vi "Destroy Texture.vi"(8 "error in (no error)":errorcluster, 11 "Texture Name":string) -> (0 "error out":errorcluster)   [LabVIEW 2021, in "Resource Manager.lvclass"]
uses:
  Resource Manager.lvclass
  Texture/Texture.lvclass
  Resource Manager.lvclass/Resource Manager.ctl
  Globals.vi
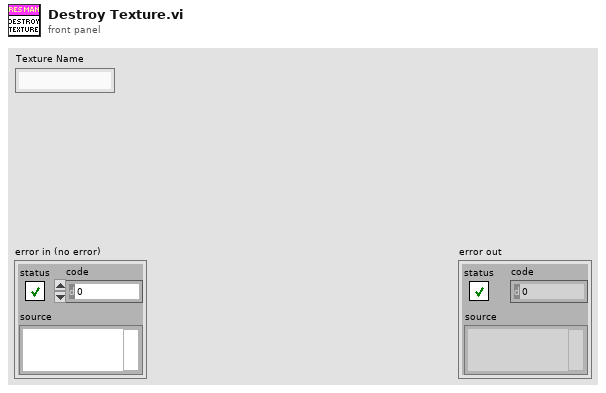
[diagram p1: front panel]
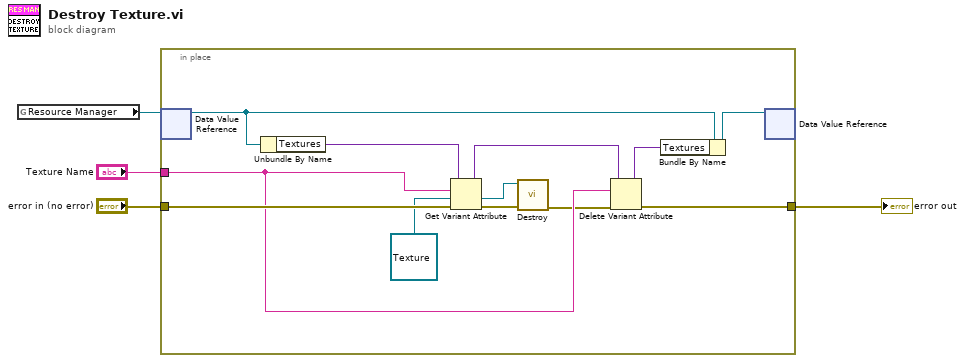
[diagram p0: block diagram]
diagram:
  n1 = global read "Globals.vi" "Resource Manager"() -> (w1:refnum<data-value>)
  n2 = in-place {
    in-place-border: "error in (no error)" -> [w15]
    in-place-border: [w12] -> w3
    in-place-border: "Texture Name" -> [w10]
    n3 = in-place-dvr #1(w1) -> (w6:refnum<class "Resource Manager.lvclass">)  [unwired: 1 out]
    n4 = Unbundle By Name(w6) -> ("Textures"=w16:variant)
    n5 = Get Variant Attribute(Variant=w16, name=w10, default value (empty Variant)=refnum<class "Texture.lvclass"> refnum ("Texture in"), error in=w15) -> (duplicate Variant=w13:variant, value=w8:refnum<class "Texture.lvclass">, error out=w9:errorcluster)  [unwired: 1 out]
    n6 = call "Destroy.vi"("error in (no error)"=w9, "Texture in"=w8) -> ("error out"=w7:errorcluster)  [unwired: 9 in]
    n7 = Delete Variant Attribute(4:w7, 6:w10, 7:w13) -> (0:w12:errorcluster, 3:w11:variant)  [unwired: 1 out]
    n8 = Bundle By Name(cluster=w6, "Textures"=w11) -> (w5:refnum<class "Resource Manager.lvclass">)
    n9 = in-place-dvr #1(w5) -> ()  [unwired: 2 out]
  }
  "error out" <- w3
